vi "even&odd.vi"() -> ()   [LabVIEW 2020]
panel:
  out "s? t:f":string
  in  "String 2":string
  in  "String":string
  out "even":bool
  in  "Numeric":dbl
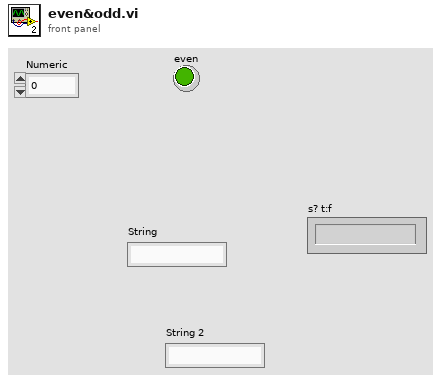
[diagram p1: front panel]
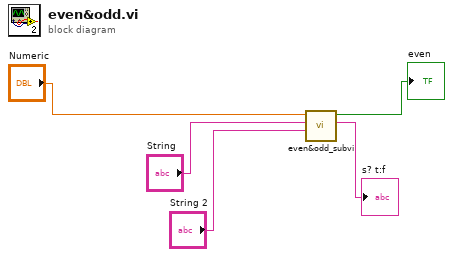
[diagram p0: block diagram]
diagram:
  n1 = call "even&odd_subvi.vi"("String 2"="String 2", "String"="String", "Numeric"="Numeric") -> ("s? t:f"=→"s? t:f":string, "even"=→"even":bool)  [unwired: 7 in]
